vi "Read from Hardware.vi"(8 "error in":errorcluster, 10 "Values in":dbl[](array[numeric]), 11 "Ballard ARINC-429 Rx Execution Unit in":refnum<class "Rx Execution Unit.lvclass">) -> (0 "error out":errorcluster, 2 "Values out":dbl[](array[numeric]), 3 "Ballard ARINC-429 Rx Execution Unit out":refnum<class "Rx Execution Unit.lvclass">)   [LabVIEW 2020, in "Ballard ARINC 429 Engine.lvlib" / "Implementation.lvlib" / "Rx Execution Unit.lvclass"]
uses:
  Rx Execution Unit.lvclass
  Execution Unit/Execution Unit.lvclass
  Custom Device/Custom Device.lvlib
  <instrlib>/BTICardLib/BTICardLV.lvlib
  Word.ctl
  Logging/Word Logging.lvlib
  C:/Dev/GitHub/niveristand-ballard-arinc429-custom-device/Source/Custom Device Support/Engine/Implementation/Execution Unit/Execution Unit.lvclass
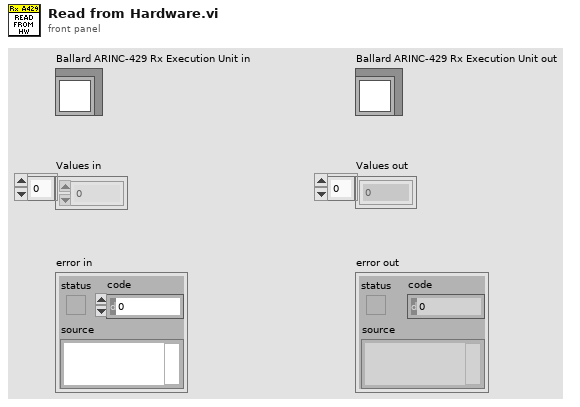
[diagram p1: front panel]
types:
  T1 = typedef "Ballard ARINC 429 Engine.lvlib/Implementation.lvlib/Word Logging.lvlib/Word.ctl" = cluster{"message info":cluster{"hardware channel":u8, "label":u8, "SDI":u8}, "data word":u32, "time stamp":dbl}
  T2 = typedef "Ballard ARINC 429 Engine.lvlib/Custom Device.lvlib/Hardware Handles.ctl" = cluster{"core handle":u64, "core reader handle":u64, "channel handles":u64[]}
  T3 = cluster{"gap":i16, "parity":i16, "long word":i16, "bit timing":i16, "timeout":i16}
  T4 = map{cluster{"hardware channel":u8, "label":u8, "SDI":u8}, cluster{"data word":u32, "time stamp":dbl}}
  T5 = typedef "BTICardLV.lvlib/429 Record.ctl" = cluster{"type":u16, "count":u16, "timestamp":u32, "msgact":u16, "decgap":u16, "data":u32, "timestamph":u32}
  T6 = cluster{"gap":bool, "parity":bool, "long word":bool, "bit timing":bool, "timeout":bool}
  T7 = cluster{"hardware channel":u8, "label":u8, "SDI":u8}
  T8 = typedef "Map of Identifiers to Indexes.ctl" = map{cluster{"Port":u8, "Label":u8, "SDI":u8}, cluster{"channel index":i32, "label index":i32, "start index":i32, "parameters":i32, "timestamp index":i32}}
  T9 = typedef "RT Hardware Channel Settings.ctl" = cluster{"channel #":u16, "channel handle":u64, "labels settings for RT":T10[]}
  T10 = typedef "RT Label Settings.ctl" = cluster{"Name":string, "xmlName":string, "label":T11, "transfer period":u32, "SDI_Enabled":bool, "SDI":u8, "parameter driver data":T12, "transfer type":T16, "has timestamp?":bool, "Label Disable/Trigger Channel Reference":T15, "Message Handle":u64, "Initialized?":bool, "Word Initial Raw Value":u32, "Label Timestamp Channel Data Reference":T17, "disabled":bool}
  T11 = typedef "Label.ctl" = u8
  T12 = typedef "RT Parameters.ctl" = cluster{"parameter definitions":T13[], "Tx parameter refs":T15[]}
  T13 = typedef "Parameter Definition.ctl" = cluster{"start index":i32, "size":i32, "encoding":T14, "signed":bool, "scale multiplier":dbl, "scale offset":dbl}
  T14 = typedef "Encoding and Decoding.lvlib/Encoding.ctl" = enum16{"BNR", "BCD", "Discrete"}
  T15 = typedef "Custom Device API.lvlib/Custom Device Item Ref.ctl" = u64
  T16 = typedef "Transfer Type.ctl" = enum16{"Scheduled", "Acyclic", "Block", "Strobe"}
  T17 = typedef "Custom Device API.lvlib/Data Reference.ctl" = i32
  T18 = cluster{"receiving":T17, "specific errors":cluster{"gap":T17, "parity":T17, "long word ":T17, "bit timing":T17, "timeout":T17}}
  T19 = cluster{"receiving":dbl, "specific errors":cluster{"gap":dbl, "parity":dbl, "long word ":dbl, "bit timing":dbl, "timeout":dbl}}
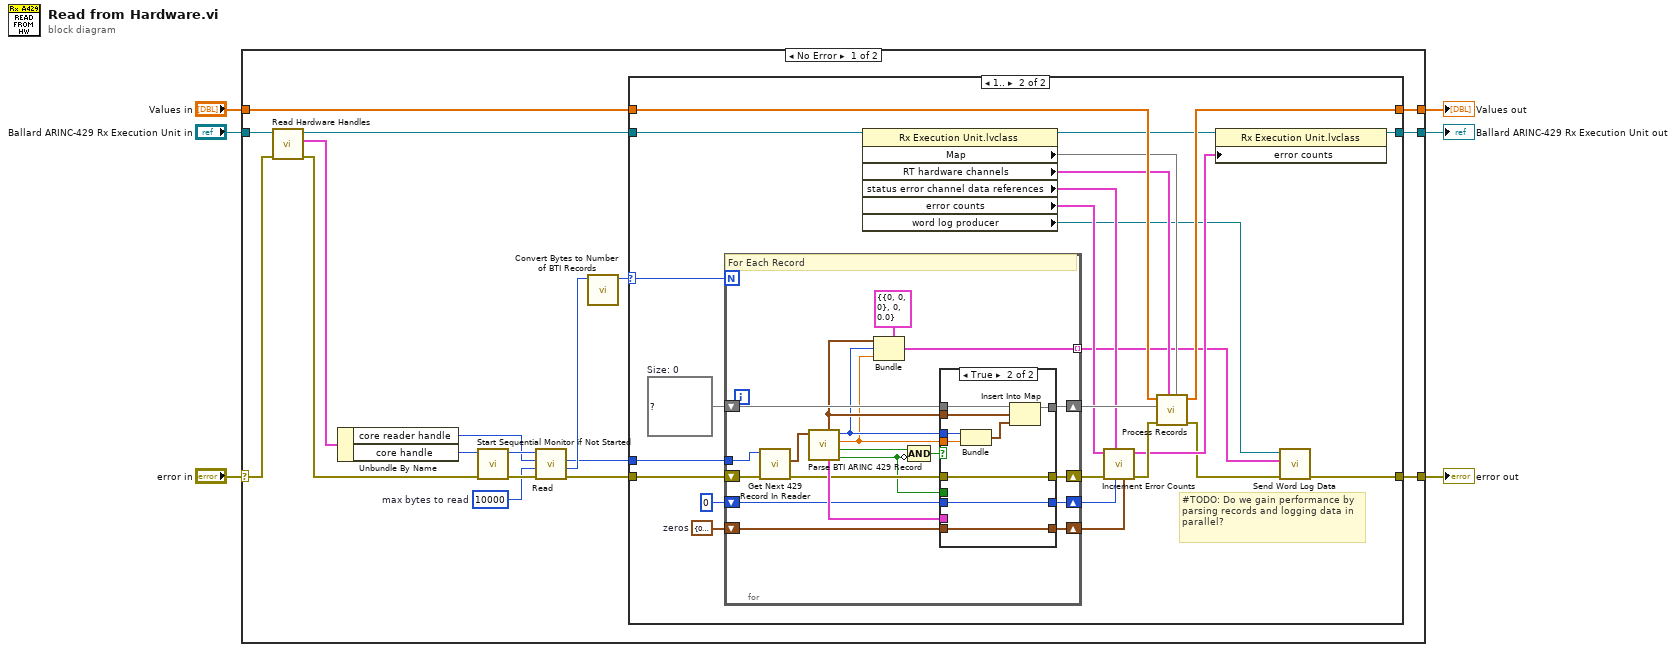
[diagram p0: block diagram]
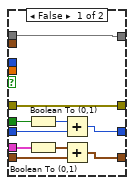
[diagram p3: hidden frame]
diagram:
  n1 = case shown="No Error" "error in" {
    selector: "error in" -> [w24 w93]
    tunnel: [w10 w94] -> w5
    tunnel: "Ballard ARINC-429 Rx Execution Unit in" -> [w23 w94]
    tunnel: [w9 w93] -> w3
    tunnel: [w8 w92] -> w2
    tunnel: "Values in" -> [w7 w92]
    frame No Error {
      w16 = 10000  # max bytes to read
      n2 = call "Read Hardware Handles.vi"("error in"=w24, "Ballard ARINC-429 Execution Unit in"=w23) -> ("error out"=w20:errorcluster, "hardware handles"=w22:T2, "Ballard ARINC-429 Execution Unit out"=w11:refnum<class "Rx Execution Unit.lvclass">)  [unwired: 7 in]
      n3 = Unbundle By Name(w22) -> ("core reader handle"=w18:u64, "core handle"=w21:u64)
      n4 = call "Start Sequential Monitor if Not Started.vi"("error in"=w20, "core handle in"=w21) -> ("error out"=w17:errorcluster, "core handle out"=w19:u64)  [unwired: 8 in]
      n5 = call <instrlib>:"Read.vi"("error in (no error)"=w17, "max bytes to read"=w16, "core reader handle in"=w18, "core handle in"=w19) -> ("error out"=w12:errorcluster, "bytes read"=w15:i32, "core reader handle out"=w13:u64)  [unwired: 4 in, 1 out]
      n6 = call "Convert Bytes to Number of BTI Records.vi"("bytes read"=w15) -> ("number of records read"=w14:i32)  [unwired: 10 in]
      n7 = case shown="1.." w14 {
        selector: w14 -> [_ w52]
        tunnel: w13 -> [_ w51]
        tunnel: w12 -> [w26 w50]
        tunnel: w11 -> [w27 w47]
        tunnel: [w27 w32] -> w10
        tunnel: [w26 w28] -> w9
        tunnel: [w25 w49] -> w8
        tunnel: w7 -> [w25 w48]
        frame Default {
        }
        frame 1.. {
          w42 = T3 {"gap"=0, "parity"=0, "long word"=0, "bit timing"=0, "timeout"=0}  # zeros
          w44 = T4 {}  # Size: 0
          # "#TODO: Do we gain performance by parsing records and logging data in parallel?"
          n8 = for {
            N: w52 -> [_]
            tunnel: w51 -> [w72]
            shift-right: [w61] -> w40
            shift-left: w50 -> [w71]
            shift-right: [w69] -> w43
            shift-left: w44 -> [w68]
            shift-right: [w67] -> w37
            shift-left: w42 -> [w66]
            shift-right: [w59] -> w38
            shift-left: i16 0 -> [w58]
            tunnel: [w53] -> w31 mode=indexing
            # "For Each Record"
            n9 = call <instrlib>:"Get Next 429 Record In Reader.vi"("error in (no error)"=w71, "core reader handle in"=w72) -> ("error out"=w62:errorcluster, "record out"=w70:T5)  [unwired: 7 in, 1 out]
            n10 = call "Parse BTI ARINC 429 Record.vi"("record"=w70) -> ("receiving error"=w60:bool, "hit"=w64:bool, "time stamp"=w54:dbl, "data word"=w55:u32, "specific errors"=w65:T6, "message info"=w56:T7)  [unwired: 5 in]
            n11 = Bundle(cluster=T1 {"message info"={"hardware channel"=0, "label"=0, "SDI"=0}, "data word"=0, "time stamp"=0.0} ("Word"), "message info"=w56, "data word"=w55, "time stamp"=w54) -> (w53:T1)
            n12 = Compound Arithmetic op=AND(w64, invert w60) -> (w63:bool)
            n13 = case shown="True" w63 {
              tunnel: w55 -> [_ w88]
              tunnel: w56 -> [_ w89]
              tunnel: [w82 w91] -> w69
              tunnel: w68 -> [w82 w90]
              tunnel: w66 -> [w80 w86]
              tunnel: [w76 w86] -> w67
              tunnel: w54 -> [_ w85]
              tunnel: w65 -> [w79 _]
              tunnel: w62 -> [w78 w84]
              tunnel: [w78 w84] -> w61
              tunnel: w60 -> [w77 _]
              tunnel: [w75 w83] -> w59
              tunnel: w58 -> [w73 w83]
              frame False {
                n14 = Boolean To (0,1)(Boolean=w77) -> (0, 1=w74:i16)
                n15 = Boolean To (0,1)(Boolean=w79) -> (0, 1=w81:T3)
                n16 = Add(x=w74, y=w73) -> (x+y=w75:i16)
                n17 = Add(x=w81, y=w80) -> (x+y=w76:T3)
              }
              frame True {
                n18 = Bundle("data word"=w88, "time stamp"=w85) -> (w87:cluster{"data word":u32, "time stamp":dbl})  [unwired: 1 in]
                n19 = Insert Into Map(map in=w90, key=w89, value=w87) -> (map out=w91:T4)  [unwired: 2 out]
              }
            }
          }
          n20 = property class="Rx Execution Unit.lvclass"(reference=w47) -> (reference out=w33:refnum<class "Rx Execution Unit.lvclass">, "Map"=w46:T8, "RT hardware channels"=w45:T9[], "status error channel data references"=w36:T18, "error counts"=w35:T19, "word log producer"=w30:refnum<class "Word Log Producer.lvclass">)  [unwired: 1 in, 1 out]
          n21 = call "Increment Error Counts.vi"("specific errors"=w37, "receiving errors"=w38, "status error channel data references"=w36, "error in"=w40, "error counts"=w35) -> ("error out"=w39:errorcluster, "error counts"=w34:T19)  [unwired: 5 in]
          n22 = call "Process Records.vi"("map from message info to indexes"=w46, "RT hardware channel data"=w45, "error in"=w39, "map from message info to data word"=w43, "parameter values in"=w48) -> ("error out"=w29:errorcluster, "parameter values out"=w49:dbl[])  [unwired: 3 in]
          n23 = property class="Rx Execution Unit.lvclass"(reference=w33, "error counts"=w34) -> (reference out=w32:refnum<class "Rx Execution Unit.lvclass">)  [unwired: 1 in, 1 out]
          n24 = call "Send Word Log Data.vi"("error in (no error)"=w29, "Data"=w31, "Producer in"=w30) -> ("error out"=w28:errorcluster)  [unwired: 7 in, 1 out]
        }
      }
    }
    frame Error {
    }
  }
  "error out" <- w3
  "Ballard ARINC-429 Rx Execution Unit out" <- w5
  "Values out" <- w2
